vi "bats.parser.test.Time.Once.vi"(10 "Expected":T2[](array[typedef])=[{"OrderBook Command.Type"=enum."Time", "Side (U8)"=0, "Order Id (U64)"=0, "Quantity (U32)"=0, "Symbol (U64)"=0, "Price (U64)"=0, "Executed Quantity (U32)"=0, "Canceled Quantity (U32)"=0, "Remaining Quantity (U32)"=0, "Seconds (U64)"=447001, "Nanoseconds (U64)"=0}] {"Side (U8)" format="%.0x"; "Order Id (U64)" format="%.0x"; "Symbol (U64)" format="%.0x"}) -> ()   [LabVIEW 2022 SP3]
uses:
  fpga/common/orderbook.command.ctl
  fpga/common/orderbook.command.type.ctl
  pitch/Time/Time.Parameters.ctl
  pitch/Time/Time.lvclass
panel:
  in  "Time.Parameters":T1={"Time"=447001}
  out "Debug":u64[](array[numeric])
  out "Passed":bool
  out "OrderBook.Command[]":T2[](array[typedef]) {"Side (U8)" format="%.0x"; "Order Id (U64)" format="%.0x"; "Symbol (U64)" format="%.0x"}
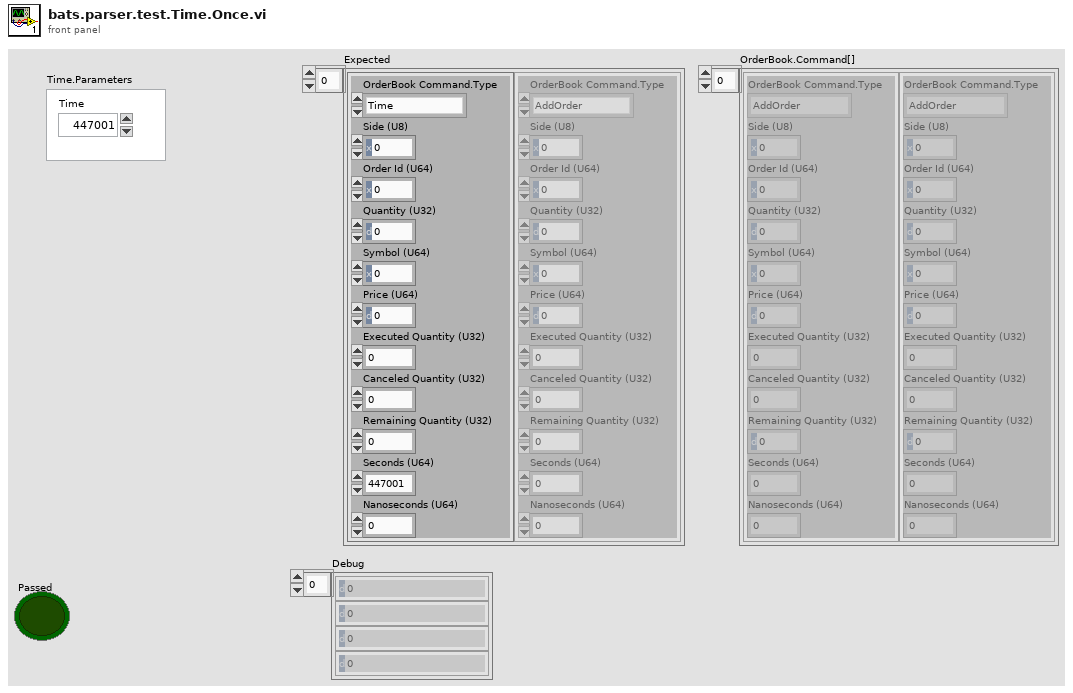
[diagram p1: front panel]
types:
  T1 = typedef "Time.lvclass/Time.Parameters.ctl" = cluster{"Time":u32}
  T2 = typedef "orderbook.command.ctl" = cluster{"OrderBook Command.Type":T3, "Side (U8)":u8, "Order Id (U64)":u64, "Quantity (U32)":u32, "Symbol (U64)":u64, "Price (U64)":u64, "Executed Quantity (U32)":u32, "Canceled Quantity (U32)":u32, "Remaining Quantity (U32)":u32, "Seconds (U64)":u64, "Nanoseconds (U64)":u64}
  T3 = typedef "orderbook.command.type.ctl" = enum16{"Time", "AddOrder", "OrderExecuted", "OrderExecutedAtPrice", "ReduceSize", "ModifyOrder", "DeleteOrder", "Get.State", "Get.All.Orders", "Get.Top"}
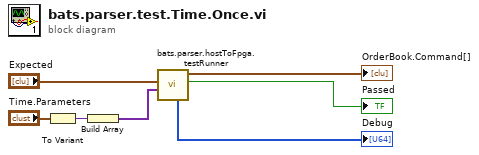
[diagram p0: block diagram]
diagram:
  n1 = To Variant(anything="Time.Parameters") -> (Variant=w2:variant)
  n2 = Build Array(w2) -> (w1:variant[])
  n3 = call "bats.parser.hostToFpga.testRunner.vi"("Test.Messages"=w1, "Expected OrderBook.Command[]"="Expected") -> ("Passed"=→"Passed":bool, "OrderBook.Command[]"=→"OrderBook.Command[]":T2[], "Debug"=→"Debug":u64[])  [unwired: 6 in, 1 out]
